vi "Set Valve Pos Impl.vi"(8 "error in (no error)":errorcluster, 10 "Valve Pos":u16, 11 "Alltesta Autosampler in":refnum<class "Alltesta Autosampler.lvclass">) -> (0 "error out":errorcluster, 3 "Alltesta Autosampler out":refnum<class "Alltesta Autosampler.lvclass">)   [LabVIEW 2023, in "Alltesta Autosampler.lvlib" / "Alltesta Autosampler.lvclass"]
uses:
  Alltesta Autosampler.lvclass
  Alltesta Autosampler.lvclass/Alltesta Autosampler.ctl
  Alltesta Autosampler.lvlib
panel:
  out "Response":string
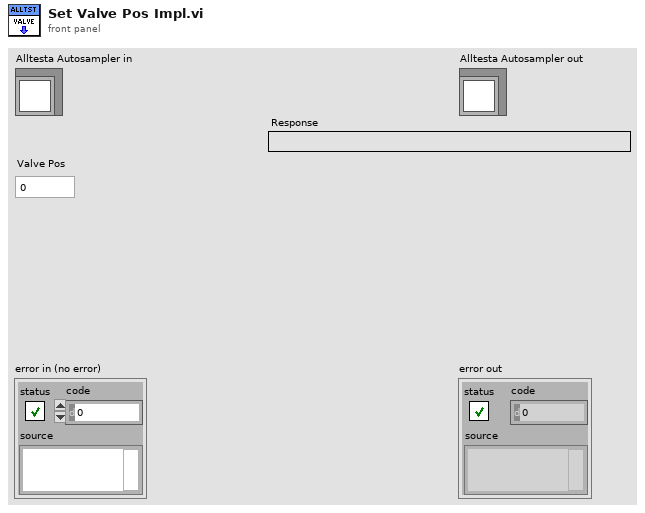
[diagram p1: front panel]
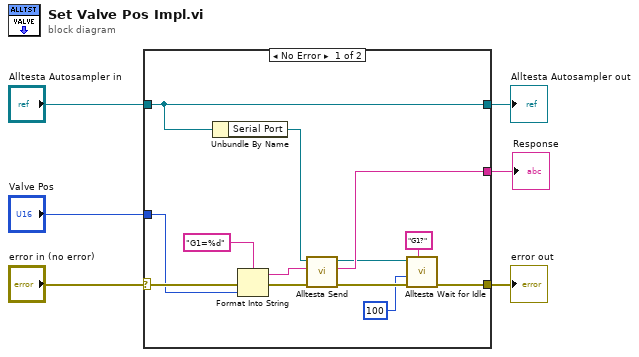
[diagram p0: block diagram]
diagram:
  n1 = case shown="No Error" "error in (no error)" {
    selector: "error in (no error)" -> [w16 w20]
    tunnel: [w7 w20] -> w5
    tunnel: "Alltesta Autosampler in" -> [w15 w21]
    tunnel: [w15 w21] -> w3
    tunnel: "Valve Pos" -> [w13 _]
    tunnel: [w12 _] -> w1
    frame No Error {
      n2 = Unbundle By Name(w15) -> ("Serial Port"=w14:refnum<visa-resource-name>)
      n3 = Format Into String(format string="G1=%d", error in=w16, w13) -> (resulting string=w19:string, error out=w18:errorcluster)  [unwired: 1 in]
      n4 = call "Alltesta Send.vi"("error in (no error)"=w18, "Command"=w19, "Serial Port in"=w14) -> ("error out"=w11:errorcluster, "Response"=w12:string, "Serial Port out"=w10:refnum<visa-resource-name>)  [unwired: 6 in]
      n5 = call "Alltesta Wait for Idle.vi"("Poll Command"="G1?", "error in (no error)"=w11, "Lower Bound"=100, "Serial Port in"=w10) -> ("error out"=w7:errorcluster)  [unwired: 6 in, 1 out]
    }
    frame Error {
    }
  }
  "error out" <- w5
  "Alltesta Autosampler out" <- w3
  "Response" <- w1
